vi "Get settings chain.vi"(8 "error in (no error)":errorcluster, 11 "TomoBase in":refnum<class "Tomo.lvclass">) -> (0 "error out":errorcluster, 1 "class name":string[](array[string]), 2 "settings":variant[](array[variant]), 3 "TomoBase out":refnum<class "Tomo.lvclass">)   [LabVIEW 2012, in "Tomo.lvclass"]
doc: "Returns an array of variants containing the settings clusters of each class in the inheritance chain (lowest child class first), together with an array of all class names in the inheritance chain.\n\nFor classes without settings cluster, the settings chain contains empty variants."
uses:
  Tomo.lvclass
  <vilib>/Distrio/Murmex/Murmex/Murmex.lvclass
  Tomo.lvclass/Tomo.ctl
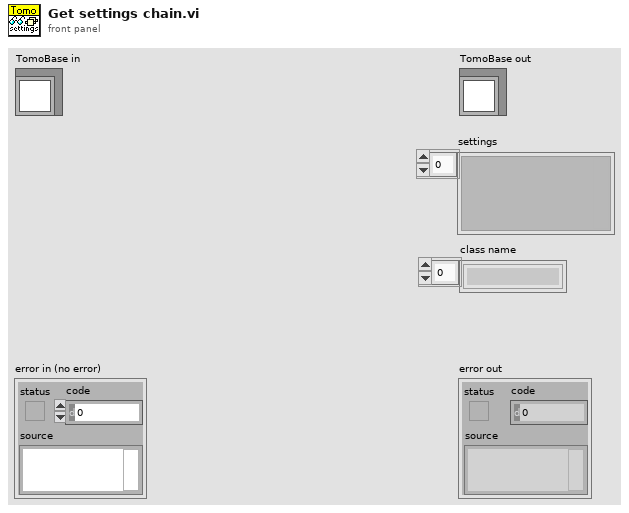
[diagram p1: front panel]
types:
  T1 = typedef "Tomo.lvclass/settings cluster.ctl" = cluster{"step sizes":cluster{"Z step size":dbl[unit], "X step size":dbl[unit], "Y step size":dbl[unit], "number of views":dbl}, "coordinates":cluster{"X min":dbl[unit], "X max":dbl[unit], "Y min":dbl[unit], "Y max":dbl[unit], "Z min":dbl[unit], "Z max":dbl[unit], "starting angle":dbl[unit]}, "Volume map":enum16{"Cubic volume", "Custom volume", "Self-generate volume"}, "experiment name":string, "custom volume path":path, "Frame rate":dbl[unit]}
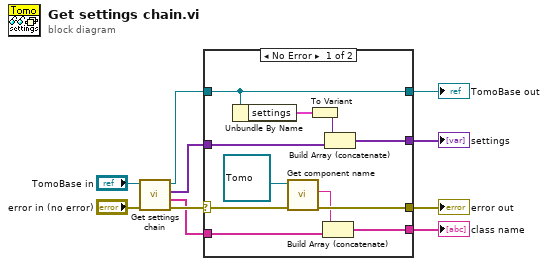
[diagram p0: block diagram]
diagram:
  n1 = call-parent "Get settings chain.vi"("error in (no error)"="error in (no error)", "MurmexBase in"="TomoBase in") -> ("error out"=w8:errorcluster, "class name"=w2:string[], "settings"=w4:variant[], "MurmexBase out"=w7:refnum<class "Tomo.lvclass">)  [unwired: 6 in]
  n2 = case shown="No Error" w8 {
    selector: w8 -> [w20 w25]
    tunnel: w7 -> [w21 w23]
    tunnel: [w21 w23] -> w6
    tunnel: [w19 w25] -> w5
    tunnel: w4 -> [w17 w24]
    tunnel: [w14 w24] -> w3
    tunnel: w2 -> [w13 w22]
    tunnel: [w11 w22] -> w1
    frame No Error {
      n3 = Unbundle By Name(w21) -> ("settings"=w16:T1)
      n4 = call <vilib>:"Get component name.vi"("error in (no error)"=w20, "Murmex in"=refnum<class "Tomo.lvclass"> refnum ("TomoBase in")) -> ("error out"=w19:errorcluster, "component name"=w12:string)  [unwired: 7 in, 1 out]
      n5 = To Variant(anything=w16) -> (Variant=w15:variant)
      n6 = Build Array (concatenate)(w12, w13) -> (w11:string[])
      n7 = Build Array (concatenate)(w15, w17) -> (w14:variant[])
    }
    frame Error {
    }
  }
  "error out" <- w5
  "TomoBase out" <- w6
  "settings" <- w3
  "class name" <- w1
